vi "P3.vi"() -> ()   [LabVIEW 2019]
panel:
  out "Array":dbl[][](array[numeric])
  out "Column Itrations":i32
  out "Row Iterations":i32
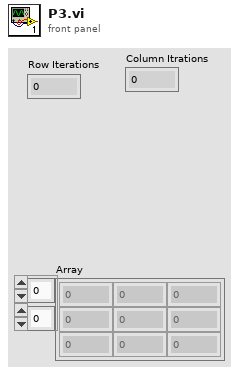
[diagram p1: front panel]
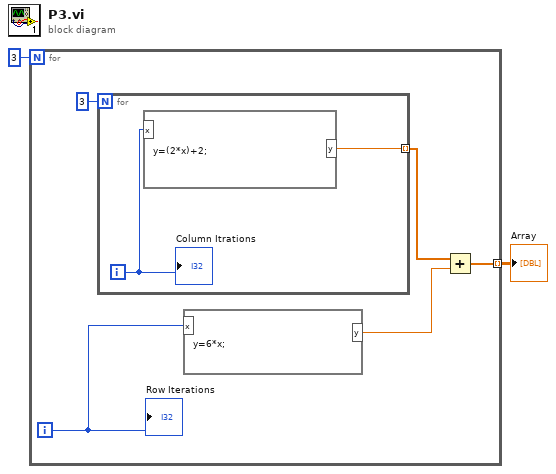
[diagram p0: block diagram]
diagram:
  n1 = for {
    N: 3 -> [_]
    tunnel: [w3] -> w1 mode=indexing
    i -> [w6]
    n2 = for {
      N: 3 -> [_]
      tunnel: [w8] -> w5 mode=indexing
      i -> [w9]
      n3 = formula code="y=(2*x)+2;"("x"=w9) -> ("y"=w8:dbl)
      "Column Itrations" <- w9
    }
    n4 = formula code="y=6*x;"("x"=w6) -> ("y"=w4:dbl)
    n5 = Add(x=w5, y=w4) -> (x+y=w3:dbl[])
    "Row Iterations" <- w6
  }
  "Array" <- w1
